vi "Error If Module Not Exist.vi"(8 "Error in":errorcluster caption="Error in (no error)", 10 "Module Exist?":bool) -> (0 "Error out":errorcluster)   [LabVIEW 2020, in "CSM-TCP-Router.lvlib"]
uses:
  CSM-TCP-Router.lvlib
panel:
  in  "module name":string
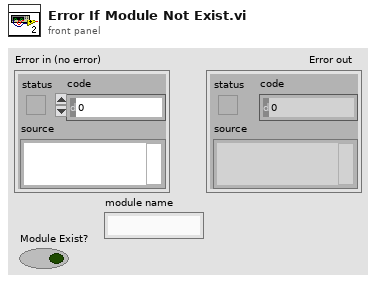
[diagram p1: front panel]
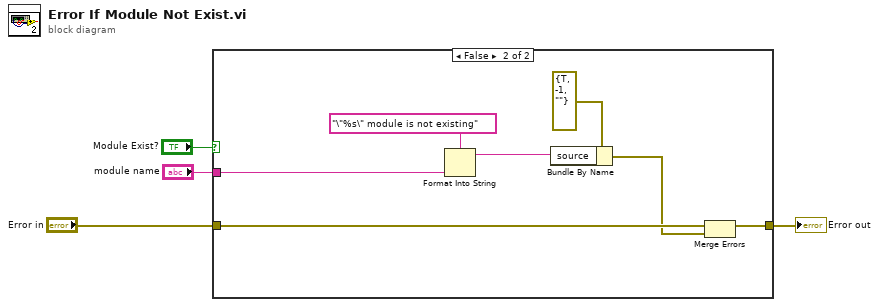
[diagram p0: block diagram]
diagram:
  n1 = case shown="False" "Module Exist?" {
    tunnel: [w5 w7] -> w3
    tunnel: "Error in" -> [w5 w8]
    tunnel: "module name" -> [_ w11]
    frame True {
    }
    frame False {
      n2 = Format Into String(format string="\"%s\" module is not existing", w11) -> (resulting string=w9:string)  [unwired: 2 in, 1 out]
      n3 = Bundle By Name(cluster=errorcluster {"status"=TRUE, "code"=-1, "source"=""} ("error in (no error)"), "source"=w9) -> (w6:errorcluster)
      n4 = Merge Errors(w8, w6) -> (w7:errorcluster)
    }
  }
  "Error out" <- w3
